vi "Find Actor Core.vi"() -> (2 "Actor Core VI Name":string, 3 "Found":bool)   [LabVIEW 2023, in "Monitored Actor.lvlib" / "Monitored Actor.lvclass"]
doc: "Looks through the call chain to find the correct version of actor core. We the Child's specific implementation of actor core if possible.\n\nBecause this will look through the call chain, this VI only works if it's run in a do method of an actor. (Not in pre-launch init for example)\n\nCopyright: MGI\n\nAuthored by Derek Trepanier\nsupport@mooregoodideas.com\nwww.mooregoodideas.com\n\nCopyright (c) 2014, Moore Good Ideas, Inc.\n\nAll rights reserved.\n\nRedistribution and use in source and binary forms, with or without modification, are permitted provided that the following conditions are met:\n\n * Redistributions of source code must retain the above copyright notice, this list of conditions and the following disclaimer.\n * Redistributions in binary form must reproduce the above copyright notice, this list of conditions and the following disclaimer in the documentation and/or other materials provided with the distribution.\n * Neither the name of Moore Good Ideas, Inc. nor the names of its contributors may be used to endorse or promote products derived from this software without specific prior written permission.\n\nTHIS SOFTWARE IS PROVIDED BY THE COPYRIGHT HOLDERS AND CONTRIBUTORS \"AS IS\" AND ANY EXPRESS OR IMPLIED WARRANTIES, INCLUDING, BUT NOT LIMITED TO, THE IMPLIED WARRANTIES OF MERCHANTABILITY AND FITNESS FOR A PARTICULAR PURPOSE ARE DISCLAIMED. IN NO EVENT SHALL THE COPYRIGHT OWNER OR CONTRIBUTORS BE LIABLE FOR ANY DIRECT, INDIRECT, INCIDENTAL, SPECIAL, EXEMPLARY, OR CONSEQUENTIAL DAMAGES (INCLUDING, BUT NOT LIMITED TO, PROCUREMENT OF SUBSTITUTE GOODS OR SERVICES; LOSS OF USE, DATA, OR PROFITS; OR BUSINESS INTERRUPTION) HOWEVER CAUSED AND ON ANY THEORY OF LIABILITY, WHETHER IN CONTRACT, STRICT LIABILITY, OR TORT (INCLUDING NEGLIGENCE OR OTHERWISE) ARISING IN ANY WAY OUT OF THE USE OF THIS SOFTWARE, EVEN IF ADVISED OF THE POSSIBILITY OF SUCH DAMAGE."
uses:
  Library/Monitored Actor.lvclass
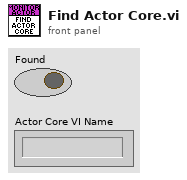
[diagram p1: front panel]
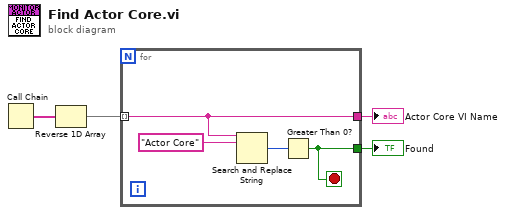
[diagram p0: block diagram]
diagram:
  n1 = Call Chain() -> (call chain=w2:string[])
  n2 = Reverse 1D Array(array=w2) -> (reversed array=w1:string[])
  n3 = for {
    tunnel: w1 -> [w5] mode=indexing
    tunnel: [w6] -> w3
    tunnel: [w5] -> w4
    stop <- w6 stop-if-true
    n4 = Search and Replace String(input string=w5, search string="Actor Core") -> (number of replacements=w7:i32)  [unwired: 6 in, 3 out]
    n5 = Greater Than 0?(x=w7) -> (x > 0?=w6:bool)
  }
  "Actor Core VI Name" <- w4
  "Found" <- w3
